vi "Variant Is LVJSON.vi"(1 "Variant":variant) -> (0 "Is LVJSON?":bool)   [LabVIEW 2019, in "labview_json.lvlib"]
uses:
  labview_json.lvlib
  <vilib>/Utility/Data Type/Type Definitions/Data Type.ctl
  <vilib>/Utility/Data Type/NI_Data Type.lvlib
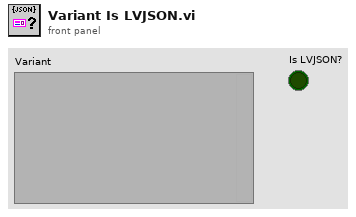
[diagram p1: front panel]
types:
  T1 = typedef "NI_Data Type.lvlib/Data Type.ctl" = enum8{"Invalid Type", "Void", "I8", "I16", "I32", "I64", "U8", "U16", "U32", "U64", "Single Float", "Double Float", "Extended Float", "Single Complex", "Double Complex", "Extended Complex", "Enum U8", "Enum U16", "Enum U32", "Enum U64", "Single Float With Unit", "Double Float With Unit", "Extended Float With Unit", "Single Complex with Unit", "Double Complex with Unit", "Extended Complex with Unit", "Boolean", "String", "Path", "Picture", "Tag", "Array", "Cluster", "Variant", "LV Variant", "Waveform", "Timestamp", "Digital Waveform", "Digital Data", "ExpressData", "Refnum", "External Data", "VI", "Poly VI", "LabVIEW Class Instance", "Fixed Point", "Set Collection", "Map Collection"}
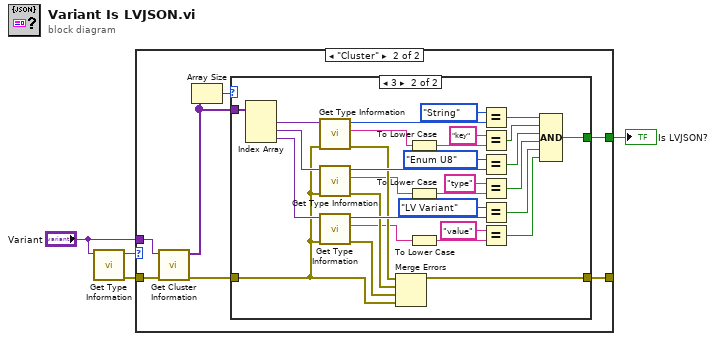
[diagram p0: block diagram]
diagram:
  n1 = call <vilib>:"Get Type Information.vi"("variant"="Variant") -> ("error out"=w4:errorcluster, "type"=w3:T1)  [unwired: 6 in, 3 out]
  n2 = case shown="\"Cluster\"" w3 {
    tunnel: "Variant" -> [_ w12]
    tunnel: [_ w9] -> w1
    tunnel: w4 -> [w5 w8]
    tunnel: [w5 w6] -> _
    frame Default {
    }
    frame "Cluster" {
      n3 = call <vilib>:"Get Cluster Information.vi"("error in (no error)"=w8, "variant"=w12) -> ("error out"=w7:errorcluster, "cluster elements"=w10:variant[])  [unwired: 8 in]
      n4 = Array Size(array=w10) -> (size(s)=w11:i32)
      n5 = case shown="3" w11 {
        tunnel: w10 -> [_ w44]
        tunnel: [_ w41] -> w9
        tunnel: w7 -> [w13 w27]
        tunnel: [w13 w40] -> w6
        frame Default {
        }
        frame 3 {
          n6 = Index Array(array=w44) -> (element #1=w32:variant, element #2=w34:variant, element #3=w35:variant)  [unwired: 3 in]
          n7 = call <vilib>:"Get Type Information.vi"("error in (no error)"=w27, "variant"=w32) -> ("error out"=w33:errorcluster, "name"=w26:string, "type"=w31:T1)  [unwired: 5 in, 2 out]
          n8 = call <vilib>:"Get Type Information.vi"("error in (no error)"=w27, "variant"=w34) -> ("error out"=w37:errorcluster, "name"=w22:string, "type"=w36:T1)  [unwired: 5 in, 2 out]
          n9 = call <vilib>:"Get Type Information.vi"("error in (no error)"=w27, "variant"=w35) -> ("error out"=w39:errorcluster, "name"=w20:string, "type"=w38:T1)  [unwired: 5 in, 2 out]
          n10 = Merge Errors(w33, w37, w39, w27) -> (w40:errorcluster)
          n11 = To Lower Case(string=w26) -> (all lower case string=w14:string)
          n12 = To Lower Case(string=w22) -> (all lower case string=w15:string)
          n13 = To Lower Case(string=w20) -> (all lower case string=w16:string)
          n14 = Equal?(x=Data_Type."String" ("Type"), y=w31) -> (x = y?=w43:bool)
          n15 = Equal?(x="key", y=w14) -> (x = y?=w24:bool)
          n16 = Equal?(x=Data_Type."Enum U8" ("Type"), y=w36) -> (x = y?=w42:bool)
          n17 = Equal?(x="type", y=w15) -> (x = y?=w19:bool)
          n18 = Equal?(x=Data_Type."LV Variant" ("Type"), y=w38) -> (x = y?=w18:bool)
          n19 = Equal?(x="value", y=w16) -> (x = y?=w17:bool)
          n20 = Compound Arithmetic op=AND(w43, w24, w42, w19, w18, w17) -> (w41:bool)
        }
      }
    }
  }
  "Is LVJSON?" <- w1
